vi "test - float.vi"(8 "error in (no error)":errorcluster, 11 "TestCase in":refnum<class "testcase-Supported-Datatype.lvclass">) -> (0 "error out":errorcluster, 3 "TestCase out":refnum<class "testcase-Supported-Datatype.lvclass">)   [LabVIEW 2017, in "testcase-Supported-Datatype.lvclass"]
uses:
  testcase-Supported-Datatype.lvclass
  56341032-296e-40a5-a01e-f46d2cc81ae2.vi
  354ad994-173a-4cf0-8e0e-293547a8b88f.vi
  e029c883-ca04-4c11-bd6f-7077957cd7a0.vi
  d683bfb0-5baf-45ce-9bbb-6c774dc2c928.vi
  a3758dbe-c78b-4687-aa2f-a1f195cd3f79.vi
  41f95f46-74a4-47e3-af3f-0ea30c484c0e.vi
  0b044080-405d-4aa6-b91a-596d98bb2048.vi
  933ab5d8-ba71-4ba5-bae6-0e686ac5fed3.vi
  addons/API-String-Arugments-Support/_Support/Data To API String Arguments.vi
  addons/API-String-Arugments-Support/_Support/Convert API String Arguments to Data(variant).vi
  <vilib>/addons/_JKI Toolkits/VI Tester/TestCase.llb/TestCase.lvclass
  C:/Program Files (x86)/National Instruments/LabVIEW 2017/vi.lib/addons/_JKI Toolkits/VI Tester/TestCase.llb/TestCase.lvclass
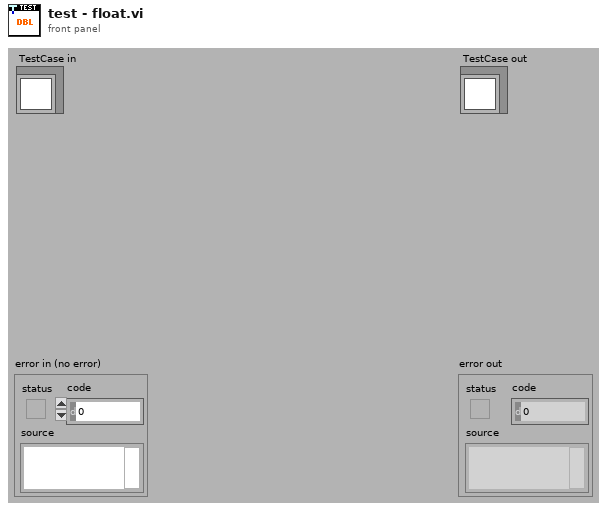
[diagram p1: front panel]
types:
  T1 = cluster{dbl, "API String":string, "Data":dbl, "error out":errorcluster}
  T2 = cluster{"string":string, "Data":dbl, "error out":errorcluster}
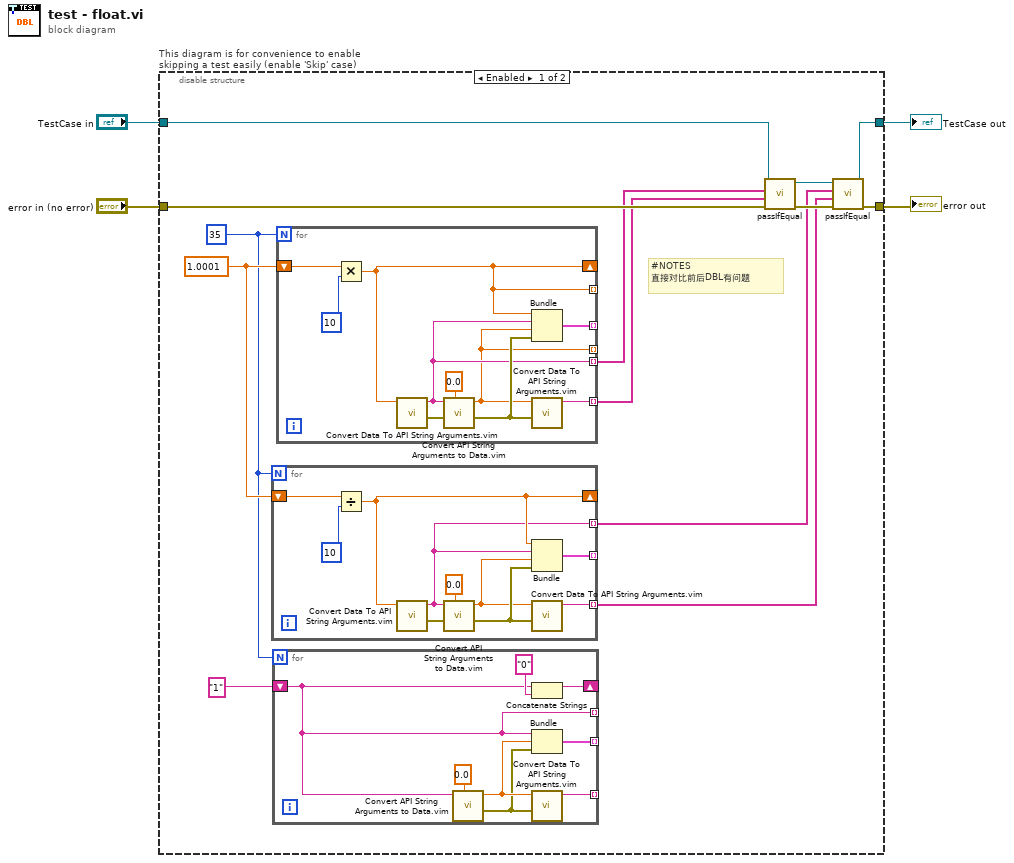
[diagram p0: block diagram]
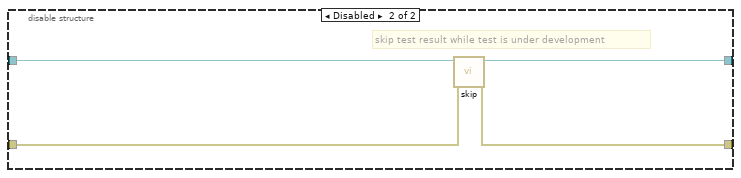
[diagram p2: hidden frame]
diagram:
  n1 = disable-structure "This diagram is for convenience to enable skipping a test easily (enable 'Skip' case)" shown="Enabled" {
    disable-tunnel: "TestCase in" -> [w17 w49]
    disable-tunnel: [w5 w47] -> w1
    disable-tunnel: [w6 w48] -> w3
    disable-tunnel: "error in (no error)" -> [w16 w46]
    frame Enabled {
      w15 = 1.0001
      w13 = 35
      # "#NOTES\n直接对比前后DBL有问题"
      n2 = for {
        N: w13 -> [_]
        shift-right: [w41] -> _
        shift-left: w15 -> [w44]
        tunnel: [w40] -> _ mode=indexing
        tunnel: [w39] -> w9 mode=indexing
        tunnel: [w36] -> w8 mode=indexing
        n3 = Divide(x=w44, y=10) -> (x/y=w41:dbl)
        n4 = call "Convert Data To API String Arguments.vim"("Data"=w41) -> ("error out"=w42:errorcluster, "API String"=w39:string)  [unwired: 7 in]
        n5 = call "Convert API String Arguments to Data.vim"("Reference Type"=0.0, "error in (no error)"=w42, "API String"=w39) -> ("error out"=w38:errorcluster, "Data"=w37:dbl)  [unwired: 5 in]
        n6 = Bundle(w41, "API String"=w39, "Data"=w37, "error out"=w38) -> (w40:T1)  [unwired: 1 in]
        n7 = call "Convert Data To API String Arguments.vim"("error in (no error)"=w38, "Data"=w37) -> ("API String"=w36:string)  [unwired: 6 in, 1 out]
      }
      n8 = for {
        N: w13 -> [_]
        shift-right: [w23] -> _
        shift-left: "1" ("string") -> [w19]
        tunnel: [w24] -> _ mode=indexing
        tunnel: [w19] -> _ mode=indexing
        tunnel: [w18] -> _ mode=indexing
        n9 = call "Convert API String Arguments to Data.vim"("Reference Type"=0.0, "API String"=w19) -> ("error out"=w20:errorcluster, "Data"=w21:dbl)  [unwired: 6 in]
        n10 = Concatenate Strings(w19, "0" ("string")) -> (w23:string)
        n11 = Bundle("string"=w19, "Data"=w21, "error out"=w20) -> (w24:T2)  [unwired: 1 in]
        n12 = call "Convert Data To API String Arguments.vim"("error in (no error)"=w20, "Data"=w21) -> ("API String"=w18:string)  [unwired: 6 in, 1 out]
      }
      n13 = for {
        N: w13 -> [_]
        shift-right: [w30] -> _
        shift-left: w15 -> [w34]
        tunnel: [w31] -> _ mode=indexing
        tunnel: [w30] -> _ mode=indexing
        tunnel: [w28] -> w11 mode=indexing
        tunnel: [w27] -> w12 mode=indexing
        tunnel: [w26] -> _ mode=indexing
        n14 = Multiply(x=w34, y=10) -> (x*y=w30:dbl)
        n15 = call "Convert Data To API String Arguments.vim"("Data"=w30) -> ("error out"=w32:errorcluster, "API String"=w27:string)  [unwired: 7 in]
        n16 = call "Convert API String Arguments to Data.vim"("Reference Type"=0.0, "error in (no error)"=w32, "API String"=w27) -> ("error out"=w29:errorcluster, "Data"=w26:dbl)  [unwired: 5 in]
        n17 = Bundle(w30, "API String"=w27, "Data"=w26, "error out"=w29) -> (w31:T1)  [unwired: 1 in]
        n18 = call "Convert Data To API String Arguments.vim"("error in (no error)"=w29, "Data"=w26) -> ("API String"=w28:string)  [unwired: 6 in, 1 out]
      }
      n19 = call-dynamic "passIfEqual.vi"("error in (no error)"=w16, "y"=w11, "x"=w12, "TestCase in"=w17) -> ("error out"=w10:errorcluster, "TestCase out"=w7:refnum<class "testcase-Supported-Datatype.lvclass">)  [unwired: 6 in]
      n20 = call-dynamic "passIfEqual.vi"("error in (no error)"=w10, "y"=w8, "x"=w9, "TestCase in"=w7) -> ("error out"=w6:errorcluster, "TestCase out"=w5:refnum<class "testcase-Supported-Datatype.lvclass">)  [unwired: 6 in]
    }
    frame Disabled {
      # "skip test result while test is under development"
      n21 = call <vilib>:"skip.vi"("error in (no error)"=w46, "TestCase in"=w49) -> ("error out"=w48:errorcluster, "TestCase out"=w47:refnum<class "testcase-Supported-Datatype.lvclass">)  [unwired: 8 in]
    }
  }
  "error out" <- w3
  "TestCase out" <- w1
